vi "ExampleMeasurementServer.vi"() -> ()   [LabVIEW 2019]
uses:
  VIs/MeasurementServer_OCVRawData.ctl
  VIs/MeasurementServer_ErrorOutData.ctl
  Global Operations.ctl
  VIs/labview-grpc-measurement-server.lvlib
panel:
  out "Cluster Time (ms)":u32
  out "OCVResults":T1[](array[typedef])=[{"battery1voltage"=0.0, "battery2voltage"=0.0, "battery3voltage"=0.0, "battery4voltage"=0.0, "battery5voltage"=0.0, "battery6voltage"=0.0, "battery7voltage"=0.0, "battery8voltage"=0.0, "battery9voltage"=0.0, "battery10voltage"=0.0, "battery11voltage"=0.0, "battery12voltage"=0.0, "battery13voltage"=0.0, "battery14voltage"=0.0, "battery15voltage"=0.0, "battery16voltage"=0.0, "battery17voltage"=0.0, "battery18voltage"=0.0, "battery19voltage"=0.0, "battery20voltage"=0.0, "battery21voltage"=0.0, "battery22voltage"=0.0, "battery23voltage"=0.0, "battery24voltage"=0.0, "ErrorOutData"={"ErrorCode"=-200220, "ErrorMessage"="DAQmx Create Channel (AI-Voltage-Basic).vi:1780001<append>\n<B>Device Specified: </B>4309_1\n<B>Suggested Device(s): </B>4309\n\n<B>Task Name: </B>_unnamedTask<8>"}}, {"battery1voltage"=0.0, "battery2voltage"=0.0, "battery3voltage"=0.0, "battery4voltage"=0.0, "battery5voltage"=0.0, "battery6voltage"=0.0, "battery7voltage"=0.0, "battery8voltage"=0.0, "battery9voltage"=0.0, "battery10voltage"=0.0, "battery11voltage"=0.0, "battery12voltage"=0.0, "battery13voltage"=0.0, "battery14voltage"=0.0, "battery15voltage"=0.0, "battery16voltage"=0.0, "battery17voltage"=0.0, "battery18voltage"=0.0, "battery19voltage"=0.0, "battery20voltage"=0.0, "battery21voltage"=0.0, "battery22voltage"=0.0, "battery23voltage"=0.0, "battery24voltage"=0.0, "ErrorOutData"={"ErrorCode"=-200220, "ErrorMessage"="DAQmx Create Channel (AI-Voltage-Basic).vi:1780001<append>\n<B>Device Specified: </B>4309_1\n<B>Suggested Device(s): </B>4309\n\n<B>Task Name: </B>_unnamedTask<8>"}}, {"battery1voltage"=0.0, "battery2voltage"=0.0, "battery3voltage"=0.0, "battery4voltage"=0.0, "battery5voltage"=0.0, "battery6voltage"=0.0, "battery7voltage"=0.0, "battery8voltage"=0.0, "battery9voltage"=0.0, "battery10voltage"=0.0, "battery11voltage"=0.0, "battery12voltage"=0.0, "battery13voltage"=0.0, "battery14voltage"=0.0, "battery15voltage"=0.0, "battery16voltage"=0.0, "battery17voltage"=0.0, "battery18voltage"=0.0, "battery19voltage"=0.0, "battery20voltage"=0.0, "battery21voltage"=0.0, "battery22voltage"=0.0, "battery23voltage"=0.0, "battery24voltage"=0.0, "ErrorOutData"={"ErrorCode"=-200220, "ErrorMessage"="DAQmx Create Channel (AI-Voltage-Basic).vi:1780001<append>\n<B>Device Specified: </B>4309_1\n<B>Suggested Device(s): </B>4309\n\n<B>Task Name: </B>_unnamedTask<8>"}}, {"battery1voltage"=0.0, "battery2voltage"=0.0, "battery3voltage"=0.0, "battery4voltage"=0.0, "battery5voltage"=0.0, "battery6voltage"=0.0, "battery7voltage"=0.0, "battery8voltage"=0.0, "battery9voltage"=0.0, "battery10voltage"=0.0, "battery11voltage"=0.0, "battery12voltage"=0.0, "battery13voltage"=0.0, "battery14voltage"=0.0, "battery15voltage"=0.0, "battery16voltage"=0.0, "battery17voltage"=0.0, "battery18voltage"=0.0, "battery19voltage"=0.0, "battery20voltage"=0.0, "battery21voltage"=0.0, "battery22voltage"=0.0, "battery23voltage"=0.0, "battery24voltage"=0.0, "ErrorOutData"={"ErrorCode"=-200220, "ErrorMessage"="DAQmx Create Channel (AI-Voltage-Basic).vi:1780001<append>\n<B>Device Specified: </B>4309_1\n<B>Suggested Device(s): </B>4309\n\n<B>Task Name: </B>_unnamedTask<8>"}}, {"battery1voltage"=0.0, "battery2voltage"=0.0, "battery3voltage"=0.0, "battery4voltage"=0.0, "battery5voltage"=0.0, "battery6voltage"=0.0, "battery7voltage"=0.0, "battery8voltage"=0.0, "battery9voltage"=0.0, "battery10voltage"=0.0, "battery11voltage"=0.0, "battery12voltage"=0.0, "battery13voltage"=0.0, "battery14voltage"=0.0, "battery15voltage"=0.0, "battery16voltage"=0.0, "battery17voltage"=0.0, "battery18voltage"=0.0, "battery19voltage"=0.0, "battery20voltage"=0.0, "battery21voltage"=0.0, "battery22voltage"=0.0, "battery23voltage"=0.0, "battery24voltage"=0.0, "ErrorOutData"={"ErrorCode"=-200220, "ErrorMessage"="DAQmx Create Channel (AI-Voltage-Basic).vi:1780001<append>\n<B>Device Specified: </B>4309_1\n<B>Suggested Device(s): </B>4309\n\n<B>Task Name: </B>_unnamedTask<8>"}}, {"battery1voltage"=0.0, "battery2voltage"=0.0, "battery3voltage"=0.0, "battery4voltage"=0.0, "battery5voltage"=0.0, "battery6voltage"=0.0, "battery7voltage"=0.0, "battery8voltage"=0.0, "battery9voltage"=0.0, "battery10voltage"=0.0, "battery11voltage"=0.0, "battery12voltage"=0.0, "battery13voltage"=0.0, "battery14voltage"=0.0, "battery15voltage"=0.0, "battery16voltage"=0.0, "battery17voltage"=0.0, "battery18voltage"=0.0, "battery19voltage"=0.0, "battery20voltage"=0.0, "battery21voltage"=0.0, "battery22voltage"=0.0, "battery23voltage"=0.0, "battery24voltage"=0.0, "ErrorOutData"={"ErrorCode"=-200220, "ErrorMessage"="DAQmx Create Channel (AI-Voltage-Basic).vi:1780001<append>\n<B>Device Specified: </B>4309_1\n<B>Suggested Device(s): </B>4309\n\n<B>Task Name: </B>_unnamedTask<8>"}}, {"battery1voltage"=0.0, "battery2voltage"=0.0, "battery3voltage"=0.0, "battery4voltage"=0.0, "battery5voltage"=0.0, "battery6voltage"=0.0, "battery7voltage"=0.0, "battery8voltage"=0.0, "battery9voltage"=0.0, "battery10voltage"=0.0, "battery11voltage"=0.0, "battery12voltage"=0.0, "battery13voltage"=0.0, "battery14voltage"=0.0, "battery15voltage"=0.0, "battery16voltage"=0.0, "battery17voltage"=0.0, "battery18voltage"=0.0, "battery19voltage"=0.0, "battery20voltage"=0.0, "battery21voltage"=0.0, "battery22voltage"=0.0, "battery23voltage"=0.0, "battery24voltage"=0.0, "ErrorOutData"={"ErrorCode"=-200220, "ErrorMessage"="DAQmx Create Channel (AI-Voltage-Basic).vi:1780001<append>\n<B>Device Specified: </B>4309_1\n<B>Suggested Device(s): </B>4309\n\n<B>Task Name: </B>_unnamedTask<8>"}}, {"battery1voltage"=0.0, "battery2voltage"=0.0, "battery3voltage"=0.0, "battery4voltage"=0.0, "battery5voltage"=0.0, "battery6voltage"=0.0, "battery7voltage"=0.0, "battery8voltage"=0.0, "battery9voltage"=0.0, "battery10voltage"=0.0, "battery11voltage"=0.0, "battery12voltage"=0.0, "battery13voltage"=0.0, "battery14voltage"=0.0, "battery15voltage"=0.0, "battery16voltage"=0.0, "battery17voltage"=0.0, "battery18voltage"=0.0, "battery19voltage"=0.0, "battery20voltage"=0.0, "battery21voltage"=0.0, "battery22voltage"=0.0, "battery23voltage"=0.0, "battery24voltage"=0.0, "ErrorOutData"={"ErrorCode"=-200220, "ErrorMessage"="DAQmx Create Channel (AI-Voltage-Basic).vi:1780001<append>\n<B>Device Specified: </B>4309_1\n<B>Suggested Device(s): </B>4309\n\n<B>Task Name: </B>_unnamedTask<8>"}}, {"battery1voltage"=0.0, "battery2voltage"=0.0, "battery3voltage"=0.0, "battery4voltage"=0.0, "battery5voltage"=0.0, "battery6voltage"=0.0, "battery7voltage"=0.0, "battery8voltage"=0.0, "battery9voltage"=0.0, "battery10voltage"=0.0, "battery11voltage"=0.0, "battery12voltage"=0.0, "battery13voltage"=0.0, "battery14voltage"=0.0, "battery15voltage"=0.0, "battery16voltage"=0.0, "battery17voltage"=0.0, "battery18voltage"=0.0, "battery19voltage"=0.0, "battery20voltage"=0.0, "battery21voltage"=0.0, "battery22voltage"=0.0, "battery23voltage"=0.0, "battery24voltage"=0.0, "ErrorOutData"={"ErrorCode"=-200220, "ErrorMessage"="DAQmx Create Channel (AI-Voltage-Basic).vi:1780001<append>\n<B>Device Specified: </B>4309_1\n<B>Suggested Device(s): </B>4309\n\n<B>Task Name: </B>_unnamedTask<8>"}}, {"battery1voltage"=0.0, "battery2voltage"=0.0, "battery3voltage"=0.0, "battery4voltage"=0.0, "battery5voltage"=0.0, "battery6voltage"=0.0, "battery7voltage"=0.0, "battery8voltage"=0.0, "battery9voltage"=0.0, "battery10voltage"=0.0, "battery11voltage"=0.0, "battery12voltage"=0.0, "battery13voltage"=0.0, "battery14voltage"=0.0, "battery15voltage"=0.0, "battery16voltage"=0.0, "battery17voltage"=0.0, "battery18voltage"=0.0, "battery19voltage"=0.0, "battery20voltage"=0.0, "battery21voltage"=0.0, "battery22voltage"=0.0, "battery23voltage"=0.0, "battery24voltage"=0.0, "ErrorOutData"={"ErrorCode"=-200220, "ErrorMessage"="DAQmx Create Channel (AI-Voltage-Basic).vi:1780001<append>\n<B>Device Specified: </B>4309_1\n<B>Suggested Device(s): </B>4309\n\n<B>Task Name: </B>_unnamedTask<8>"}}]
  in  "# of Measurements":i32=10
  out "Config Time (ms)":u32
  out "Read Time (ms)":u32
  in  "error in (no error)":errorcluster
  in  "Server Key File (.key)":path
  in  "Server Certificate File (.crt)":path
  in  "stop":bool
  in  "Server Address":string="0.0.0.0:50051"
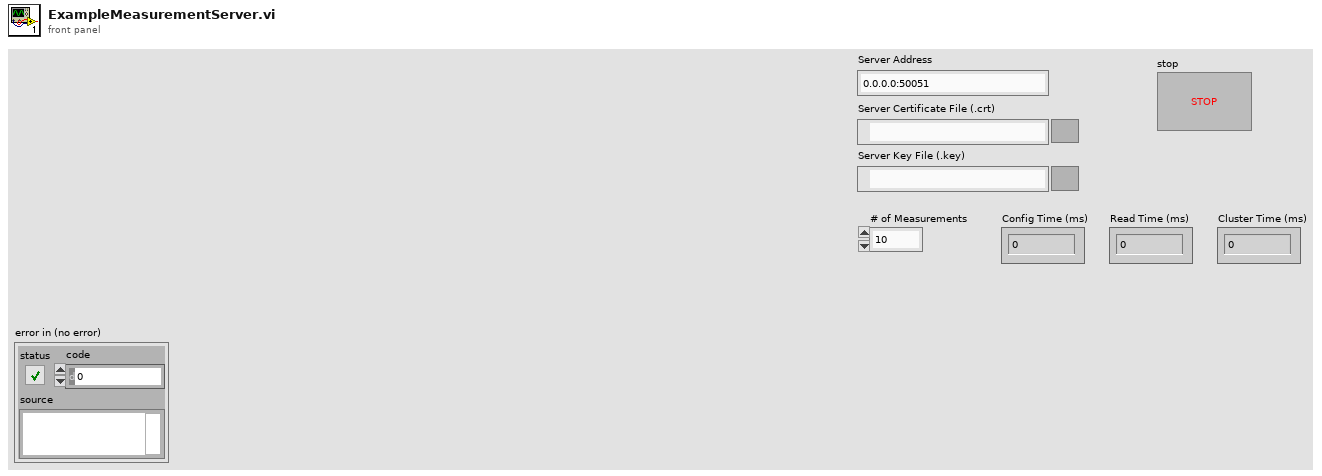
[diagram p1: front panel]
types:
  T1 = typedef "labview-grpc-measurement-server.lvlib/MeasurementServer_OCVRawData.ctl" = cluster{"battery1voltage":sgl, "battery2voltage":sgl, "battery3voltage":sgl, "battery4voltage":sgl, "battery5voltage":sgl, "battery6voltage":sgl, "battery7voltage":sgl, "battery8voltage":sgl, "battery9voltage":sgl, "battery10voltage":sgl, "battery11voltage":sgl, "battery12voltage":sgl, "battery13voltage":sgl, "battery14voltage":sgl, "battery15voltage":sgl, "battery16voltage":sgl, "battery17voltage":sgl, "battery18voltage":sgl, "battery19voltage":sgl, "battery20voltage":sgl, "battery21voltage":sgl, "battery22voltage":sgl, "battery23voltage":sgl, "battery24voltage":sgl, "ErrorOutData":T2}
  T2 = typedef "labview-grpc-measurement-server.lvlib/MeasurementServer_ErrorOutData.ctl" = cluster{"ErrorCode":i32, "ErrorMessage":string}
  T3 = typedef "labview-grpc-measurement-server.lvlib/MeasurementServer_gRPCid.ctl" = u64
  T4 = cluster{"QueryServer_Invoke":refnum<user-event>, "QueryServer_Query":refnum<user-event>, "QueryServer_Register":refnum<user-event>, "QueryServer_OCVMeasurement":refnum<user-event>, "QueryServer_StreamOCVMeasurement":refnum<user-event>, "gRPCid":T3}
  T5 = typedef "Global Operations.ctl" = enum16{"Get", "Set"}
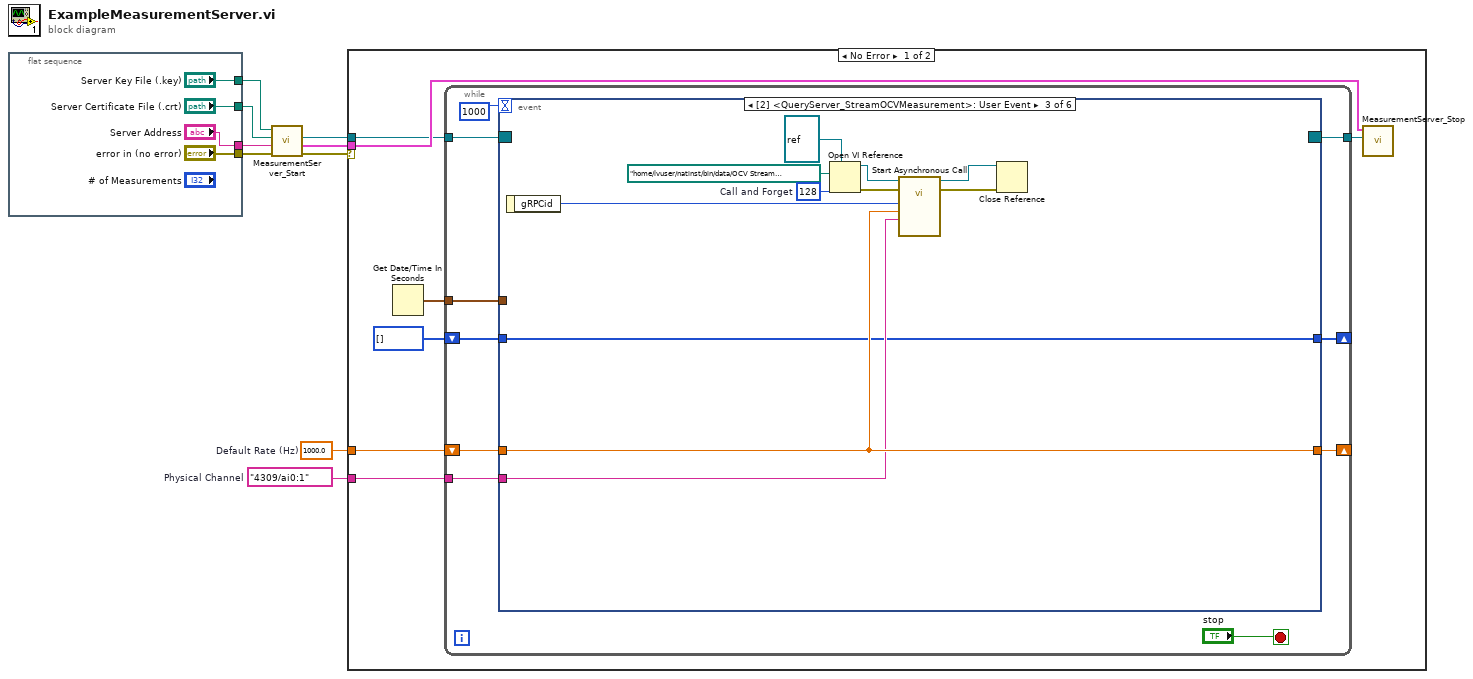
[diagram p0: block diagram]
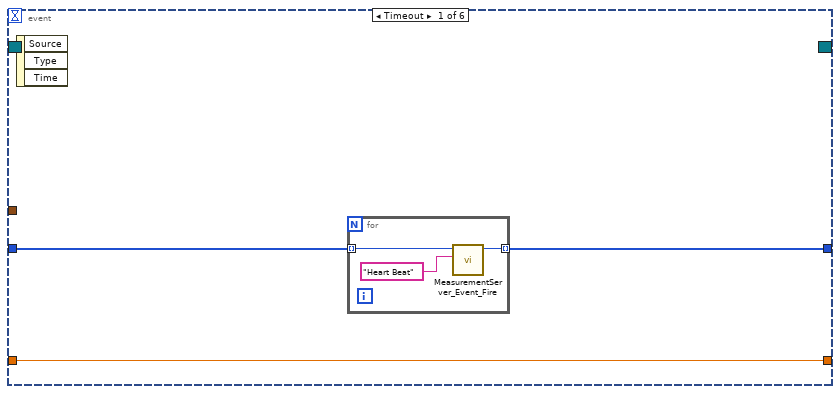
[diagram p2: hidden frame]
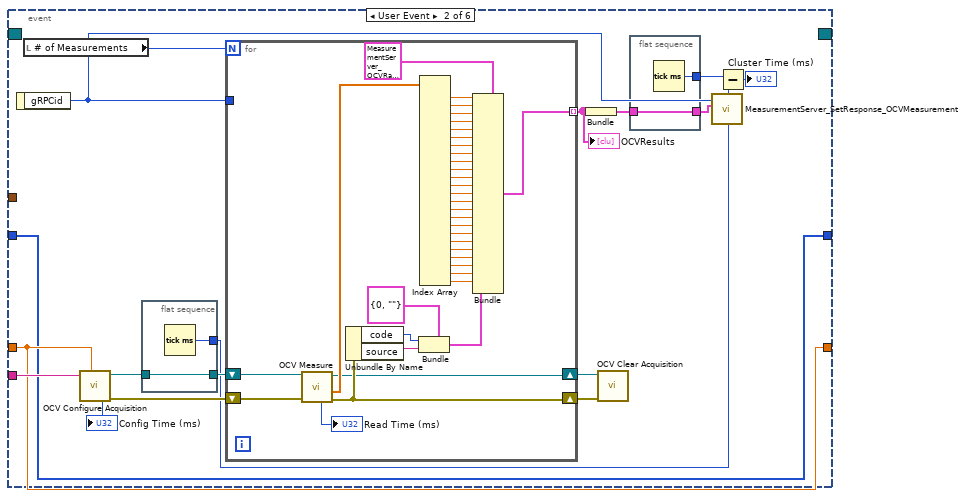
[diagram p3: hidden frame]
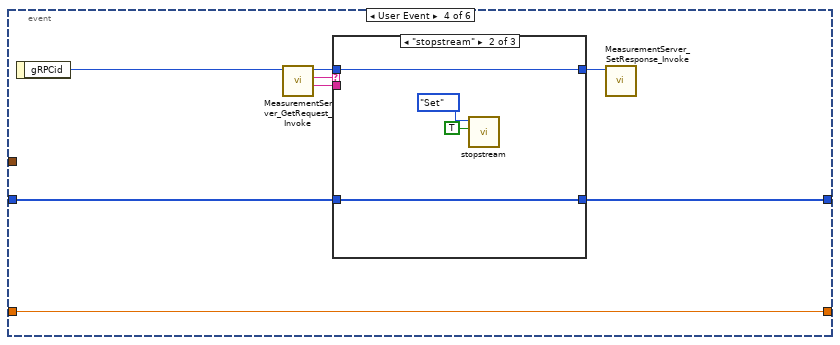
[diagram p4: hidden frame]
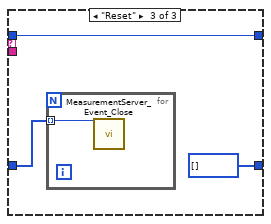
[diagram p6: hidden frame]
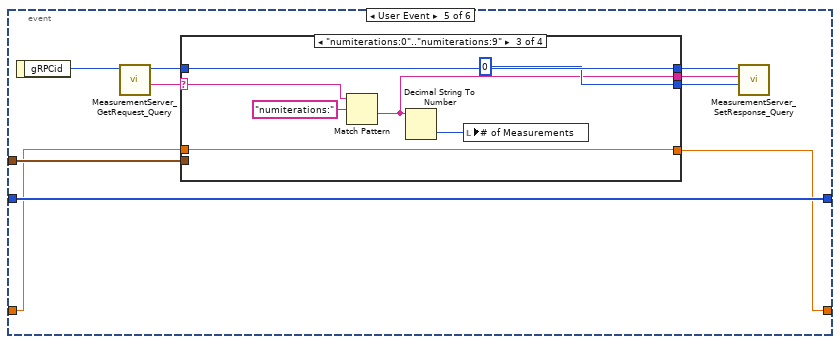
[diagram p7: hidden frame]
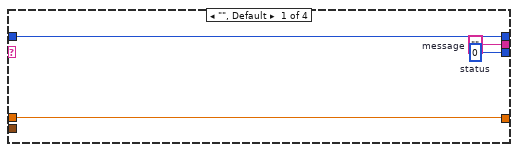
[diagram p8: hidden frame]
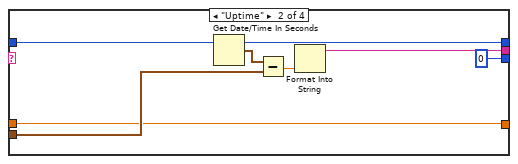
[diagram p9: hidden frame]
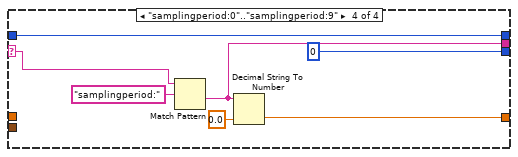
[diagram p10: hidden frame]
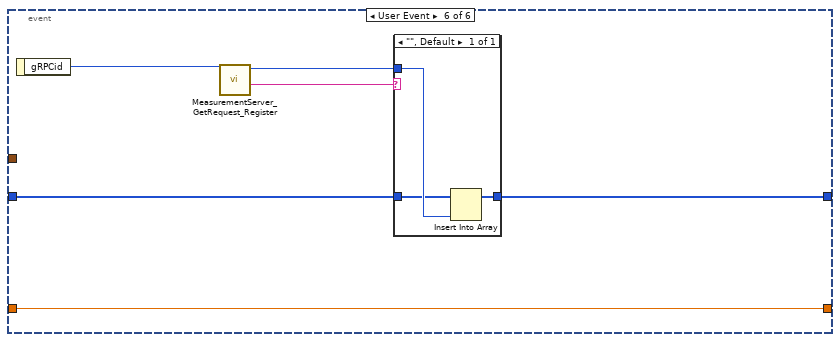
[diagram p11: hidden frame]
diagram:
  w2 = tag "4309/ai0:1"  # Physical Channel
  w1 = 1000.0  # Default Rate (Hz)
  n1 = flat-sequence {
    tunnel: ["error in (no error)"] -> w9
    tunnel: ["Server Key File (.key)"] -> w6
    tunnel: ["Server Certificate File (.crt)"] -> w5
    tunnel: ["Server Address"] -> w4
    frame #0 {
    }
  }
  n2 = call "MeasurementServer_Start.vi"("error in (no error)"=w9, "Server Address"=w4, "Server Certificate File (.crt)"=w5, "Server Key File (.key)"=w6) -> ("error out"=w3:errorcluster, "Cluster"=w7:T4, "Event Registration Ref"=w8:refnum<event-registration>)  [unwired: 4 in, 1 out]
  n3 = case shown="No Error" w3 {
    tunnel: w7 -> [w18 _]
    tunnel: w8 -> [w17 _]
    tunnel: w2 -> [w15 _]
    tunnel: w1 -> [w14 _]
    frame No Error {
      n4 = Get Date/Time In Seconds() -> (seconds since 1Jan1904=w20:timestamp)
      n5 = while {
        tunnel: w20 -> [w29]
        shift-right: [w27] -> _
        shift-left: u64[] [] -> [w26]
        tunnel: w17 -> [w25]
        tunnel: [w24] -> w16
        tunnel: w15 -> [w23]
        shift-right: [w21] -> _
        shift-left: w14 -> [w22]
        stop <- "stop" stop-if-true
        n6 = event shown="[2] <QueryServer_StreamOCVMeasurement>: User Event" {
          selector: w25 -> [_ _ _ _ _ _]
          dyn-events: [_ _ _ _ _ _] -> w24
          timeout: 1000 -> [_ _ _ _ _ _]
          tunnel: w29 -> [_ _ _ _ w127 _]
          tunnel: [w33 w37 w94 w106 w126 w161] -> w27
          tunnel: w26 -> [w32 w37 w94 w107 w126 w160]
          tunnel: w23 -> [_ w39 w97 _ _ _]
          tunnel: w22 -> [w31 w38 w98 w105 w123 w158]
          tunnel: [w31 w38 w98 w105 w124 w158] -> w21
          event Timeout {
            n7 = event-data() -> ()  [unwired: 1 in, 3 out]
            n8 = for {
              tunnel: w32 -> [w36] mode=indexing
              tunnel: [w34] -> w33 mode=indexing
              n9 = call "MeasurementServer_Event_Fire.vi"("eventdata"="Heart Beat", "gRPCid"=w36) -> ("gRPCid out"=w34:T3)  [unwired: 8 in, 1 out]
            }
          }
          event User Event {
            n10 = event-data() -> ("gRPCid"=w53:T3)  [unwired: 1 in]
            n11 = local read "# of Measurements"() -> (w47:i32)
            n12 = call "OCV Configure Acquisition.vi"("Rate (Hz)"=w38, "Physical Channel"=w39) -> ("error out"=w48:errorcluster, "Refnum out"=w40:refnum<k21>, "Config Time"=→"Config Time (ms)":u32)  [unwired: 7 in]
            n13 = flat-sequence {
              tunnel: w40 -> [w57]
              tunnel: [w57] -> w46
              tunnel: [w56] -> w42
              frame #0 {
                n14 = Tick Count (ms)() -> (millisecond timer value=w56:u32)
              }
            }
            n15 = for {
              N: w47 -> [_]
              tunnel: w53 -> [_]
              tunnel: [w83] -> w52 mode=indexing
              shift-right: [w80] -> w51
              shift-left: w46 -> [w78]
              shift-right: [w81] -> w50
              shift-left: w48 -> [w77]
              n16 = call "OCV Measure.vi"("error in (no error)"=w77, "Refnum in"=w78) -> ("error out"=w81:errorcluster, "Voltage"=w82:sgl[], "Refnum out"=w80:refnum<k21>, "Read Time (ms)"=→"Read Time (ms)":u32)  [unwired: 6 in]
              n17 = Unbundle By Name(w81) -> ("code"=w92:i32, "source"=w91:string)
              n18 = Bundle(cluster=T2 {"ErrorCode"=0, "ErrorMessage"=""} ("ErrorOutData"), "ErrorCode"=w92, "ErrorMessage"=w91) -> (w90:T2)
              n19 = Index Array(array=w82) -> (element #1=w89:sgl, element #2=w88:sgl, element #3=w87:sgl, element #4=w86:sgl, element #5=w85:sgl, element #6=w76:sgl, element #7=w75:sgl, element #8=w74:sgl, element #9=w73:sgl, element #10=w72:sgl, element #11=w71:sgl, element #12=w70:sgl, element #13=w69:sgl, element #14=w68:sgl, element #15=w67:sgl, element #16=w66:sgl, element #17=w65:sgl, element #18=w64:sgl, element #19=w63:sgl, element #20=w62:sgl, element #21=w61:sgl, element #22=w60:sgl, element #23=w59:sgl, element #24=w58:sgl)  [unwired: 24 in]
              n20 = Bundle(cluster=T1 {"battery1voltage"=0.0, "battery2voltage"=0.0, "battery3voltage"=0.0, "battery4voltage"=0.0, "battery5voltage"=0.0, "battery6voltage"=0.0, "battery7voltage"=0.0, "battery8voltage"=0.0, "battery9voltage"=0.0, "battery10voltage"=0.0, "battery11voltage"=0.0, "battery12voltage"=0.0, "battery13voltage"=0.0, "battery14voltage"=0.0, "battery15voltage"=0.0, "battery16voltage"=0.0, "battery17voltage"=0.0, "battery18voltage"=0.0, "battery19voltage"=0.0, "battery20voltage"=0.0, "battery21voltage"=0.0, "battery22voltage"=0.0, "battery23voltage"=0.0, "battery24voltage"=0.0, "ErrorOutData"={"ErrorCode"=0, "ErrorMessage"=""}} ("OCVRawData"), "battery1voltage"=w89, "battery2voltage"=w88, "battery3voltage"=w87, "battery4voltage"=w86, "battery5voltage"=w85, "battery6voltage"=w76, "battery7voltage"=w75, "battery8voltage"=w74, "battery9voltage"=w73, "battery10voltage"=w72, "battery11voltage"=w71, "battery12voltage"=w70, "battery13voltage"=w69, "battery14voltage"=w68, "battery15voltage"=w67, "battery16voltage"=w66, "battery17voltage"=w65, "battery18voltage"=w64, "battery19voltage"=w63, "battery20voltage"=w62, "battery21voltage"=w61, "battery22voltage"=w60, "battery23voltage"=w59, "battery24voltage"=w58, "ErrorOutData"=w90) -> (w83:T1)
            }
            "OCVResults" <- w52
            n21 = Bundle(w52) -> (w45:cluster{T1[]})  [unwired: 1 in]
            n22 = call "OCV Clear Acquisition.vi"("error in (no error)"=w50, "Refnum in"=w51) -> ()  [unwired: 8 in, 2 out]
            n23 = flat-sequence {
              tunnel: w45 -> [w55]
              tunnel: [w55] -> w44
              tunnel: [w54] -> w43
              frame #0 {
                n24 = Tick Count (ms)() -> (millisecond timer value=w54:u32)
              }
            }
            n25 = call "MeasurementServer_SetResponse_OCVMeasurement.vi"("gRPCid"=w53, "OCVResponse"=w44) -> ()  [unwired: 8 in, 1 out]
            n26 = Subtract(x=w43, y=w42) -> (x-y=→"Cluster Time (ms)":u32)
          }
          event User Event {
            w103 = 128  # Call and Forget
            n27 = event-data() -> ("gRPCid"=w99:T3)  [unwired: 1 in]
            n28 = Open VI Reference(type specifier VI Refnum (for type only)=refnum<vi> refnum, vi path=path "/home/lvuser/natinst/bin/data/OCV Stream Asynchronous.vi", options=w103) -> (vi reference=w101:refnum<vi>, error out=w100:errorcluster)  [unwired: 3 in]
            n29 = call-by-ref "Start Asynchronous Call"(reference=w101, error in=w100, "Physical Channel"=w97, "Rate (Hz)"=w98, "gRPCid"=w99) -> (reference out=w96:refnum<vi>, error out=w95:errorcluster)  [unwired: 8 in, 1 out]
            n30 = Close Reference(reference=w96, error in (no error)=w95) -> ()  [unwired: 1 out]
          }
          event User Event {
            n31 = event-data() -> ("gRPCid"=w112:T3)  [unwired: 1 in]
            n32 = call "MeasurementServer_GetRequest_Invoke.vi"("gRPCid"=w112) -> ("parameter"=w108:string, "command"=w111:string, "gRPCid out"=w110:T3)  [unwired: 5 in, 1 out]
            n33 = case shown="\"stopstream\"" w111 {
              tunnel: w110 -> [w114 w118 w119]
              tunnel: [w114 w118 w119] -> w109
              tunnel: w108 -> [_ _ _]
              tunnel: w107 -> [w113 w117 w121]
              tunnel: [w113 w117 u64[] []] -> w106
              frame "", Default {
              }
              frame "stopstream" {
                n34 = call "stopstream.vi"("STOPSTREAM"=TRUE, "Operation"=Global_Operations."Set") -> ()  [unwired: 8 in, 2 out]
              }
              frame "Reset" {
                n35 = for {
                  tunnel: w121 -> [w122] mode=indexing
                  n36 = call "MeasurementServer_Event_Close.vi"("gRPCid"=w122) -> ()  [unwired: 9 in, 1 out]
                }
              }
            }
            n37 = call "MeasurementServer_SetResponse_Invoke.vi"("gRPCid"=w109) -> ()  [unwired: 9 in, 1 out]
          }
          event User Event {
            n38 = event-data() -> ("gRPCid"=w132:T3)  [unwired: 1 in]
            n39 = call "MeasurementServer_GetRequest_Query.vi"("gRPCid"=w132) -> ("gRPCid out"=w131:T3, "query"=w125:string)  [unwired: 7 in, 1 out]
            n40 = case shown="\"numiterations:0\"..\"numiterations:9\"" w125 {
              selector: w125 -> [_ _ w148 w155]
              tunnel: w131 -> [w136 w140 w150 w157]
              tunnel: [w136 w140 w150 w157] -> w130
              tunnel: [w135 w141 w145 w153] -> w129
              tunnel: [w134 0 ("status") 0 ("status") 0 ("status")] -> w128
              tunnel: w127 -> [_ w138 _ _]
              tunnel: [w133 w137 w144 w151] -> w124
              tunnel: w123 -> [w133 w137 w144 _]
              frame "", Default {
                w134 = 0  # status
                w135 = ""  # message
              }
              frame "Uptime" {
                n41 = Get Date/Time In Seconds() -> (seconds since 1Jan1904=w143:timestamp)
                n42 = Subtract(x=w143, y=w138) -> (x-y=w142:dbl)
                n43 = Format Into String(w142) -> (resulting string=w141:string)  [unwired: 3 in, 1 out]
              }
              frame "numiterations:0".."numiterations:9" {
                n44 = Match Pattern(string=w148, regular expression="numiterations:") -> (after substring=w145:string)  [unwired: 1 in, 3 out]
                n45 = Decimal String To Number(string=w145) -> (number=w146:i32)  [unwired: 2 in, 1 out]
                n46 = local write "# of Measurements"(w146) -> ()
              }
              frame "samplingperiod:0".."samplingperiod:9" {
                n47 = Match Pattern(string=w155, regular expression="samplingperiod:") -> (after substring=w153:string)  [unwired: 1 in, 3 out]
                n48 = Decimal String To Number(string=w153, default (0L)=0.0 ("Rate (Hz)")) -> (number=w151:dbl)  [unwired: 1 in, 1 out]
              }
            }
            n49 = call "MeasurementServer_SetResponse_Query.vi"("gRPCid"=w130, "message"=w129, "status"=w128) -> ()  [unwired: 7 in, 1 out]
          }
          event User Event {
            n50 = event-data() -> ("gRPCid"=w163:T3)  [unwired: 1 in]
            n51 = call "MeasurementServer_GetRequest_Register.vi"("gRPCid"=w163) -> ("gRPCid out"=w162:T3, "eventname"=w159:string)  [unwired: 7 in, 1 out]
            n52 = case shown="\"\", Default" w159 {
              tunnel: w162 -> [w166]
              tunnel: [w165] -> w161
              tunnel: w160 -> [w164]
              frame "", Default {
                n53 = Insert Into Array(array=w164, new element=w166) -> (w165:T3[])  [unwired: 1 in]
              }
            }
          }
        }
      }
      n54 = call "MeasurementServer_Stop.vi"("Server Information"=w18, "Event Registration Refnum"=w16) -> ()  [unwired: 8 in, 1 out]
    }
    frame Error {
    }
  }
